vi "Launcher prueba.vi"   [LabVIEW 2020]
uses:
  Binary counter.lvclass
  C:/Program Files/National Instruments/LabVIEW 2020/vi.lib/ActorFramework/Actor/Actor.lvclass
  <vilib>/ActorFramework/Actor/Actor.lvclass
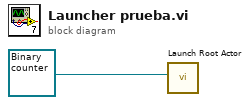
[diagram p0: block diagram]
diagram:
  n1 = call <vilib>:"Launch Root Actor.vi"("Actor"=refnum<class "Binary counter.lvclass"> refnum ("Binary counter.lvlib:Binary counter.lvclass")) -> ()  [unwired: 9 in, 2 out]
